vi "setFPGAReference.vi"(10 "FPGAReference":refnum<k20>, 11 "MyHealthAndStatusReadFIFO in":refnum<class "ModbusPort2ReadFIFO.lvclass">) -> (3 "MyHealthAndStatusReadFIFO out":refnum<class "ModbusPort2ReadFIFO.lvclass">)   [LabVIEW 2015, in "ModbusPort2ReadFIFO.lvclass"]
uses:
  ModbusPort2ReadFIFO.lvclass
  ModbusPort2ReadFIFO.lvclass/ModbusPort2ReadFIFO.ctl
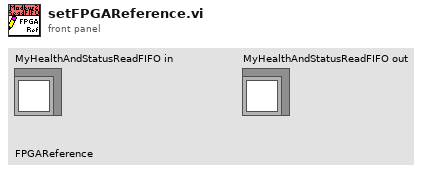
[diagram p1: front panel]
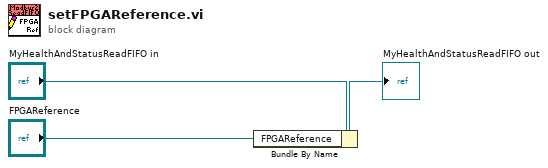
[diagram p0: block diagram]
diagram:
  n1 = Bundle By Name(cluster="MyHealthAndStatusReadFIFO in", "FPGAReference"="FPGAReference") -> (→"MyHealthAndStatusReadFIFO out":refnum<class "ModbusPort2ReadFIFO.lvclass">)
